vi "Test DB_CONNECTOR API.vi"() -> ()   [LabVIEW 2014]
doc: "DB_CONNECTOR API Tester.\n\n____\nHAMPEL SOFTWARE ENGINEERING v2.4.4 (2020-05-26 17:37)"
uses:
  Query Poly-VIs/Query - String - 2D.vi
  DB_CONNECTOR.lvlib
panel:
  out "DB-Type":string
  in  "Get DB-Type":bool
  in  "btn_Fast_Query":bool caption="btn_Query"
  out "Query Time (ms)":u32
  out "Field Names":string[](array[string])
  in  "Config Section":string
  out "Meta Data":variant
  in  "btn_Commit_Transaction":bool caption="btn_Query"
  in  "btn_Start_Transaction":bool caption="btn_Query"
  out "Return Data":string[][](array[string])
  in  "btn_Query":bool
  in  "SQL Query":string
  in  "Run as Singleton?":bool
  in  "Show Block Diagram":bool
  in  "Refresh Modules":bool
  out "Active Modules":string[](array[string])
  in  "Stop Module":bool
  in  "Select Module":i32(ring)=-1 caption="Select Module\nTo send Request to" items=["All"=-1]
  in  "Run New Module":bool
  in  "Hide Module Panel":bool
  in  "Show Module Panel":bool
  out "Status":string
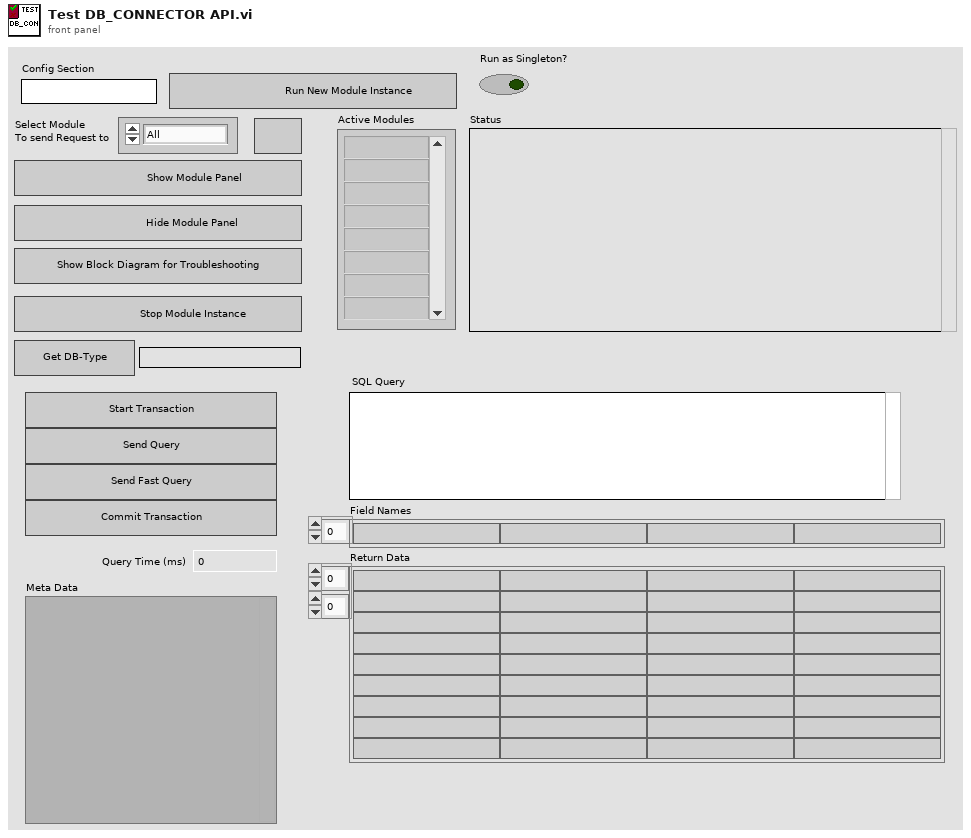
[diagram p1: front panel]
types:
  T1 = typedef "DB_CONNECTOR.lvlib/Broadcast Events--cluster.ctl" = cluster{"Module Did Init":refnum<user-event>, "Status Updated":refnum<user-event>, "Error Reported":refnum<user-event>, "Module Did Stop":refnum<user-event>, "Update Module Execution Status":refnum<user-event>, "Fast Query Reply":refnum<user-event>}
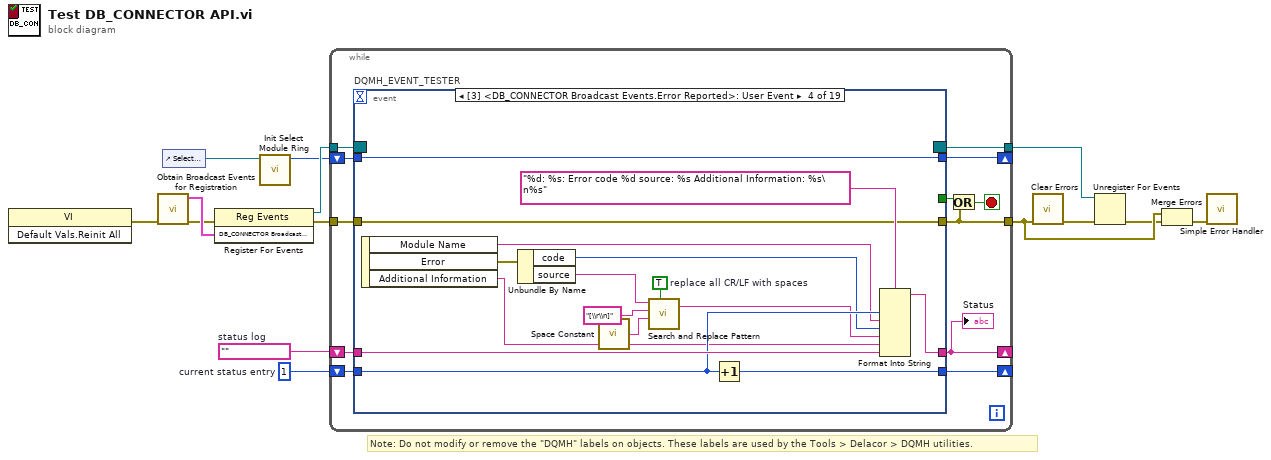
[diagram p0: block diagram]
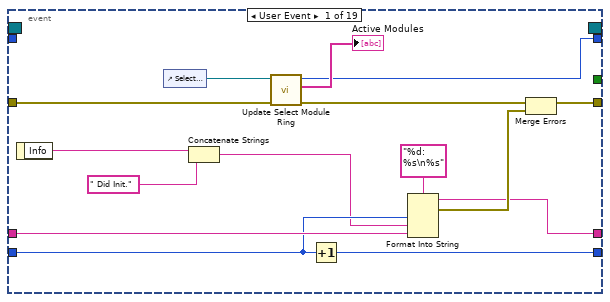
[diagram p2: hidden frame]
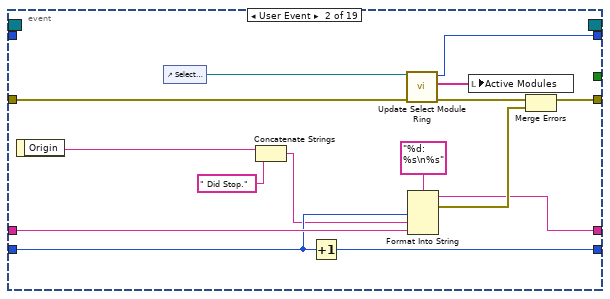
[diagram p3: hidden frame]
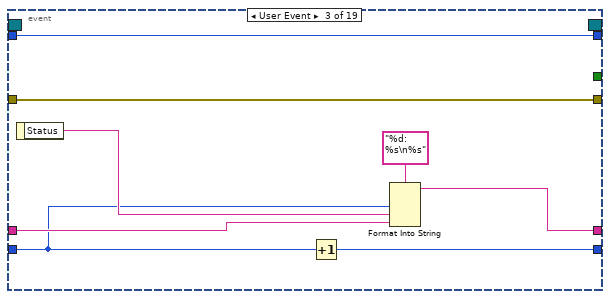
[diagram p4: hidden frame]
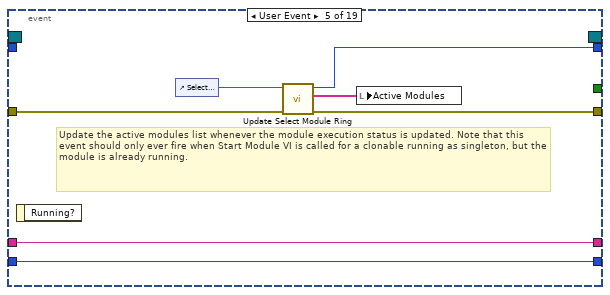
[diagram p5: hidden frame]
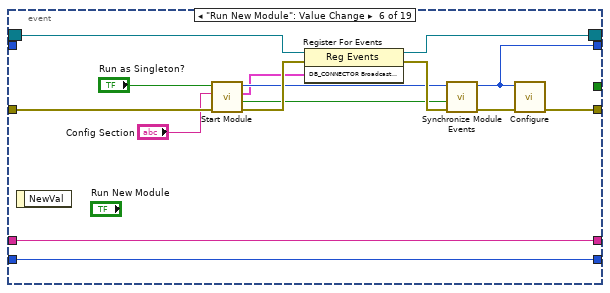
[diagram p6: hidden frame]
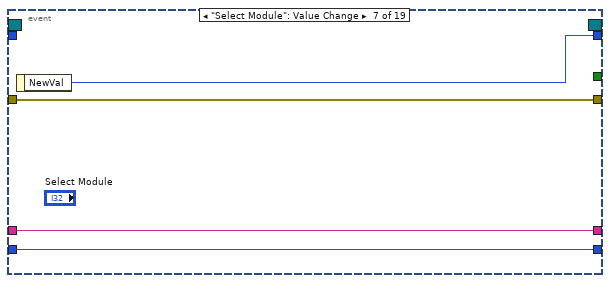
[diagram p7: hidden frame]
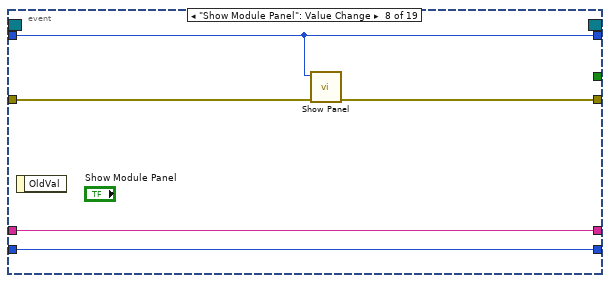
[diagram p8: hidden frame]
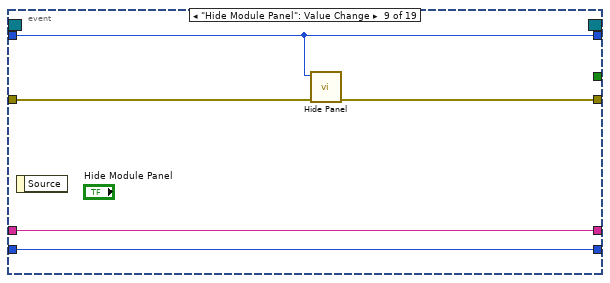
[diagram p9: hidden frame]
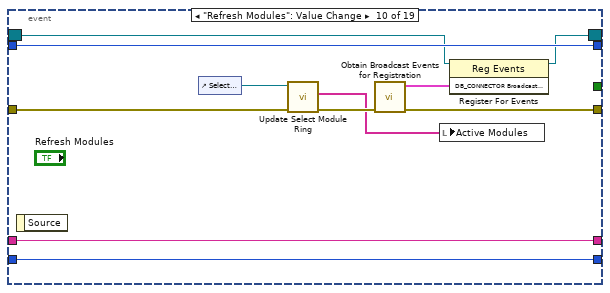
[diagram p10: hidden frame]
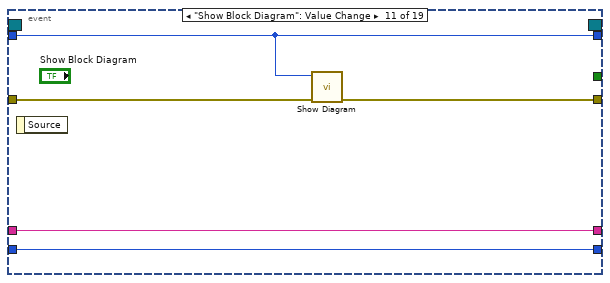
[diagram p11: hidden frame]
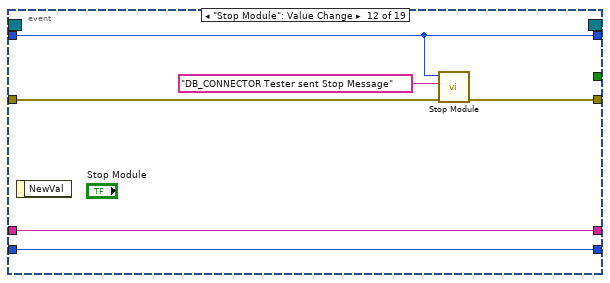
[diagram p12: hidden frame]
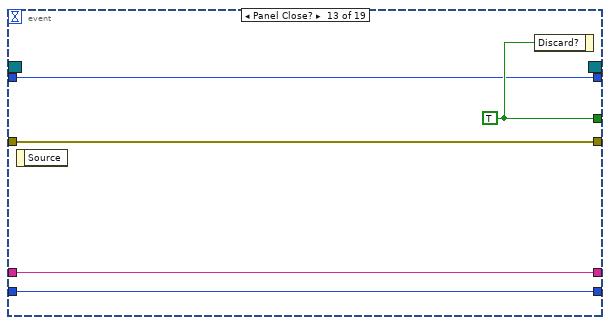
[diagram p13: hidden frame]
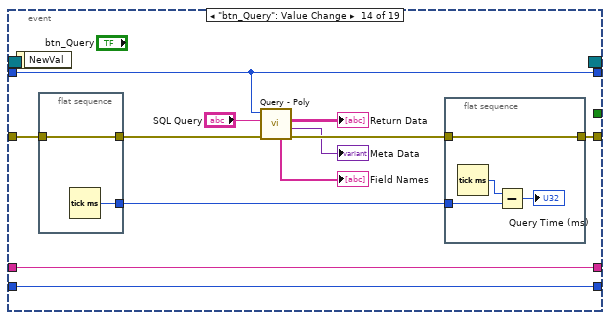
[diagram p14: hidden frame]
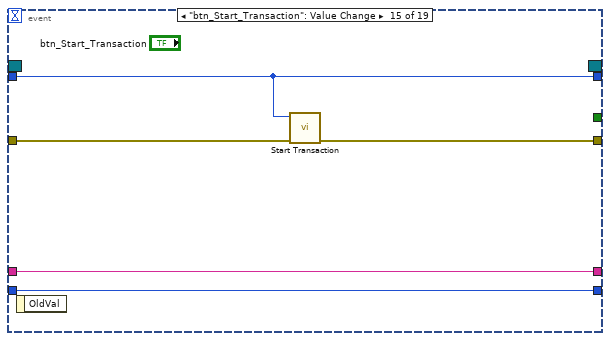
[diagram p15: hidden frame]
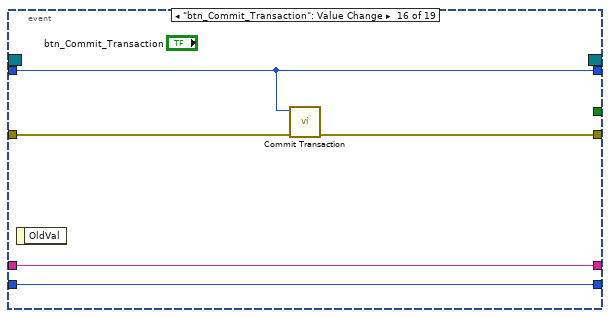
[diagram p16: hidden frame]
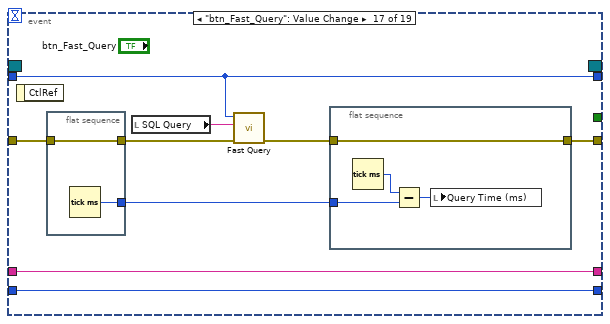
[diagram p17: hidden frame]
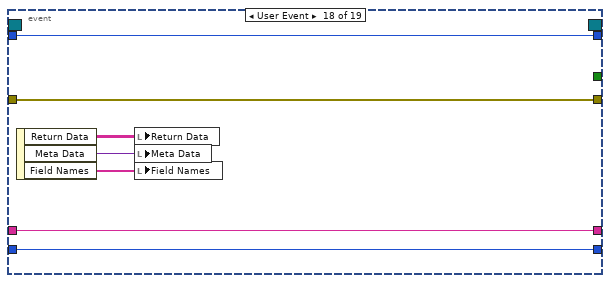
[diagram p18: hidden frame]
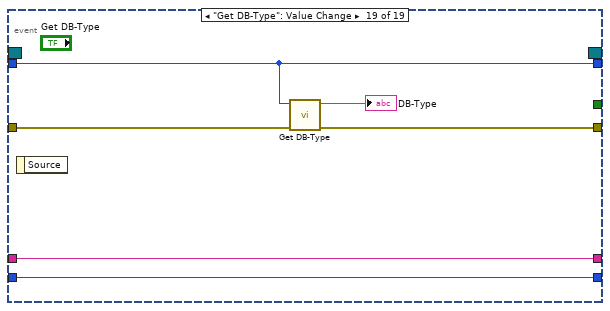
[diagram p19: hidden frame]
diagram:
  w11 = 1  # current status entry
  w12 = ""  # status log
  # "Note: Do not modify or remove the \"DQMH\" labels on objects. These labels are used by the Tools > Delacor > DQMH utilities."
  n1 = invoke class="VI" method="Default Vals.Reinit All"() -> (error out=w3:errorcluster)  [unwired: 3 in, 2 out]
  n2 = call "Obtain Broadcast Events for Registration.vi"("error in (no error)"=w3) -> ("error out"=w2:errorcluster, "DB_CONNECTOR Broadcast Events"=w8:T1)  [unwired: 9 in]
  n3 = control-ref of="Select Module"() -> (w9:refnum<vi>)
  n4 = register-events(error in=w2, w8) -> (reference out=w14:refnum<event-registration>, error out=w7:errorcluster)  [unwired: 1 in]
  n5 = call "Init Select Module Ring.vi"("Select Module Ring Ref"=w9) -> ("Value for All Modules"=w10:i32)  [unwired: 8 in, 2 out]
  n6 = while {
    tunnel: w14 -> [w26]
    tunnel: [w15] -> w4
    tunnel: w7 -> [w24]
    shift-right: [w20] -> _
    shift-left: w12 -> [w22]
    shift-right: [w21] -> _
    shift-left: w11 -> [w23]
    shift-right: [w17] -> _
    shift-left: w10 -> [w18]
    tunnel: [w16] -> w6
    stop <- w19 stop-if-true
    n7 = event "DQMH_EVENT_TESTER" shown="[3] <DB_CONNECTOR Broadcast Events.Error Reported>: User Event" {
      selector: w26 -> [_ _ _ _ _ w97 _ _ _ w122 _ _ _ _ _ _ _ _ _]
      dyn-events: [_ _ _ _ _ w96 _ _ _ w121 _ _ _ _ _ _ _ _ _] -> w16
      timeout: _ -> [_ _ _ _ _ _ _ _ _ _ _ _ _ _ _ _ _ _ _]
      tunnel: [_ _ _ _ _ _ _ _ _ _ _ _ w143 _ _ _ _ _ _] -> w25
      tunnel: [w30 w48 w64 w70 w83 w90 w106 w110 w115 w118 w129 w134 w142 w145 w163 w168 w173 w193 w196] -> w15
      tunnel: w24 -> [w32 w50 w64 w70 w84 w98 w106 w111 w116 w123 w132 w135 w142 w147 w166 w171 w176 w193 w199]
      tunnel: w23 -> [w38 w53 w57 w76 w86 w99 w104 w108 w113 w126 w130 w137 w140 w153 w164 w169 w179 w191 w197]
      tunnel: w22 -> [w39 w54 w60 w78 w87 w100 w105 w109 w114 w127 w131 w138 w141 w154 w165 w170 w180 w192 w198]
      tunnel: [w36 w51 w61 w73 w87 w100 w105 w109 w114 w127 w131 w138 w141 w154 w165 w170 w180 w192 w198] -> w20
      tunnel: [w37 w52 w63 w79 w86 w99 w104 w108 w113 w126 w130 w137 w140 w153 w164 w169 w179 w191 w197] -> w21
      tunnel: w18 -> [_ _ w58 w80 _ _ _ w107 w112 w125 w128 w136 w139 w152 w162 w167 w178 w190 w195]
      tunnel: [w27 w45 w58 w80 w82 w89 w103 w107 w112 w125 w128 w136 w139 w152 w162 w167 w178 w190 w195] -> w17
      event User Event {
        n8 = event-data() -> ("Info"=w35:string)  [unwired: 1 in]
        n9 = control-ref of="Select Module"() -> (w29:refnum<vi>)
        n10 = Concatenate Strings(w35, " Did Init.") -> (w34:string)
        n11 = call "Update Select Module Ring.vi"("error in (no error)"=w32, "Select Module Ring Ref"=w29) -> ("error out"=w31:errorcluster, "Active Modules (Array)"=→"Active Modules":string[], "New Module Ring Value"=w27:i32)  [unwired: 7 in]
        n12 = Increment(x=w38) -> (x+1=w37:i32)
        n13 = Format Into String(format string="%d: %s\n%s", w38, w34, w39) -> (resulting string=w36:string, error out=w41:errorcluster)  [unwired: 2 in]
        n14 = Merge Errors(w31, w41) -> (w30:errorcluster)
      }
      event User Event {
        n15 = event-data() -> ("Origin"=w43:string)  [unwired: 1 in]
        n16 = control-ref of="Select Module"() -> (w47:refnum<vi>)
        n17 = Concatenate Strings(w43, " Did Stop.") -> (w42:string)
        n18 = Increment(x=w53) -> (x+1=w52:i32)
        n19 = call "Update Select Module Ring.vi"("error in (no error)"=w50, "Select Module Ring Ref"=w47) -> ("error out"=w49:errorcluster, "Active Modules (Array)"=w46:string[], "New Module Ring Value"=w45:i32)  [unwired: 7 in]
        n20 = Format Into String(format string="%d: %s\n%s", w53, w42, w54) -> (resulting string=w51:string, error out=w56:errorcluster)  [unwired: 2 in]
        n21 = local write "Active Modules"(w46) -> ()
        n22 = Merge Errors(w49, w56) -> (w48:errorcluster)
      }
      event User Event {
        n23 = event-data() -> ("Status"=w59:string)  [unwired: 1 in]
        n24 = Increment(x=w57) -> (x+1=w63:i32)
        n25 = Format Into String(format string="%d: %s\n%s", w57, w59, w60) -> (resulting string=w61:string)  [unwired: 2 in, 1 out]
      }
      event User Event {
        w74 = TRUE  # replace all CR/LF with spaces
        n26 = event-data() -> ("Module Name"=w68:string, "Error"=w67:errorcluster, "Additional Information"=w65:string)  [unwired: 1 in]
        n27 = Unbundle By Name(w67) -> ("code"=w69:i32, "source"=w71:string)
        n28 = call <vilib>:"Space Constant.vi"() -> ("String"=w75:string)
        n29 = call <vilib>:"Search and Replace Pattern.vi"("string"=w71, "regular expression (\"\")"="[\\r\\n]" ("regular expression (\"\")"), "replace string (\"\")"=w75, "replace all? (F)"=w74) -> ("result string"=w72:string)  [unwired: 1 in, 1 out]
        n30 = Increment(x=w76) -> (x+1=w79:i32)
        n31 = Format Into String(format string="%d: %s: Error code %d source: %s Additional Information: %s\n%s", w76, w68, w69, w72, w65, w78) -> (resulting string=w73:string)  [unwired: 2 in, 1 out]
      }
      event User Event {
        # "Update the active modules list whenever the module execution status is updated. Note that this event should only ever fire when Start Module VI is called for a clonable running as singleton, but the module is already running."
        n32 = event-data() -> ()  [unwired: 1 in, 1 out]
        n33 = control-ref of="Select Module"() -> (w85:refnum<vi>)
        n34 = call "Update Select Module Ring.vi"("error in (no error)"=w84, "Select Module Ring Ref"=w85) -> ("error out"=w83:errorcluster, "Active Modules (Array)"=w81:string[], "New Module Ring Value"=w82:i32)  [unwired: 7 in]
        n35 = local write "Active Modules"(w81) -> ()
      }
      event "Run New Module": Value Change {
        n36 = event-data() -> ()  [unwired: 1 in, 1 out]
        n37 = call "Start Module.vi"("error in (no error)"=w98, "Config Section"="Config Section", "Run as Singleton? (F)"="Run as Singleton?") -> ("error out"=w101:errorcluster, "Wait for Event Sync?"=w94:bool, "DB_CONNECTOR Broadcast Events"=w93:T1, "Module ID"=w95:i32)  [unwired: 5 in]
        n38 = register-events(reference=w97, error in=w101, w93) -> (reference out=w96:refnum<event-registration>, error out=w102:errorcluster)
        n39 = call "Synchronize Module Events.vi"("error in (no error)"=w102, "Wait for Event Sync?"=w94, "Module ID"=w95) -> ("error out"=w91:errorcluster, "Module ID (dup)"=w89:i32)  [unwired: 7 in]
        n40 = call "Configure.vi"("error in (no error)"=w91, "Module ID"=w89) -> ("error out"=w90:errorcluster)  [unwired: 8 in, 1 out]
      }
      event "Select Module": Value Change {
        n41 = event-data() -> ("NewVal"=w103:i32)  [unwired: 1 in]
      }
      event "Show Module Panel": Value Change {
        n42 = event-data() -> ()  [unwired: 1 in, 1 out]
        n43 = call "Show Panel.vi"("error in (no error)"=w111, "Module ID"=w107) -> ("error out"=w110:errorcluster)  [unwired: 9 in]
      }
      event "Hide Module Panel": Value Change {
        n44 = event-data() -> ()  [unwired: 1 in, 1 out]
        n45 = call "Hide Panel.vi"("error in (no error)"=w116, "Module ID"=w112) -> ("error out"=w115:errorcluster)  [unwired: 9 in]
      }
      event "Refresh Modules": Value Change {
        n46 = event-data() -> ()  [unwired: 1 in, 1 out]
        n47 = control-ref of="Select Module"() -> (w124:refnum<vi>)
        n48 = call "Update Select Module Ring.vi"("error in (no error)"=w123, "Select Module Ring Ref"=w124) -> ("error out"=w119:errorcluster, "Active Modules (Array)"=w117:string[])  [unwired: 7 in, 1 out]
        n49 = call "Obtain Broadcast Events for Registration.vi"("error in (no error)"=w119) -> ("error out"=w118:errorcluster, "DB_CONNECTOR Broadcast Events"=w120:T1)  [unwired: 9 in]
        n50 = local write "Active Modules"(w117) -> ()
        n51 = register-events(reference=w122, w120) -> (reference out=w121:refnum<event-registration>)  [unwired: 1 in, 1 out]
      }
      event "Show Block Diagram": Value Change {
        n52 = event-data() -> ()  [unwired: 1 in, 1 out]
        n53 = call "Show Diagram.vi"("error in (no error)"=w132, "Module ID"=w128) -> ("error out"=w129:errorcluster)  [unwired: 9 in]
      }
      event "Stop Module": Value Change {
        n54 = event-data() -> ()  [unwired: 1 in, 1 out]
        n55 = call "Stop Module.vi"("error in (no error)"=w135, "Origin"="DB_CONNECTOR Tester sent Stop Message", "Module ID"=w136) -> ("error out"=w134:errorcluster)  [unwired: 8 in]
      }
      event Panel Close? {
        w143 = TRUE ("Discard?")
        n56 = event-data() -> ()  [unwired: 1 in, 1 out]
        n57 = event-data("Discard?"=w143) -> ()  [unwired: 1 in, 1 out]
      }
      event "btn_Query": Value Change {
        n58 = event-data() -> ()  [unwired: 1 in, 1 out]
        n59 = flat-sequence {
          tunnel: w147 -> [w161]
          tunnel: [w161] -> w146
          tunnel: [w160] -> w144
          frame #0 {
            n60 = Tick Count (ms)() -> (millisecond timer value=w160:u32)
          }
        }
        n61 = call-poly "Query - Poly.vi"("error in"=w146, "Query"="SQL Query", "Module ID"=w152) -> ("error out"=w155:errorcluster, "Meta Data"=→"Meta Data":variant, "Return Data"=→"Return Data":string[][], "Field Names"=→"Field Names":string[])  [unwired: 5 in]
        n62 = flat-sequence {
          tunnel: w155 -> [w159]
          tunnel: [w159] -> w145
          tunnel: w144 -> [w157]
          frame #0 {
            n63 = Tick Count (ms)() -> (millisecond timer value=w158:u32)
            n64 = Subtract(x=w158, y=w157) -> (x-y=→"Query Time (ms)":u32)
          }
        }
      }
      event "btn_Start_Transaction": Value Change {
        n65 = event-data() -> ()  [unwired: 1 in, 1 out]
        n66 = call "Start Transaction.vi"("error in (no error)"=w166, "Module ID"=w162) -> ("error out"=w163:errorcluster)  [unwired: 9 in]
      }
      event "btn_Commit_Transaction": Value Change {
        n67 = event-data() -> ()  [unwired: 1 in, 1 out]
        n68 = call "Commit Transaction.vi"("error in (no error)"=w171, "Module ID"=w167) -> ("error out"=w168:errorcluster)  [unwired: 7 in, 2 out]
      }
      event "btn_Fast_Query": Value Change {
        n69 = event-data() -> ()  [unwired: 1 in, 1 out]
        n70 = flat-sequence {
          tunnel: w176 -> [w186]
          tunnel: [w186] -> w175
          tunnel: [w185] -> w172
          frame #0 {
            n71 = Tick Count (ms)() -> (millisecond timer value=w185:u32)
          }
        }
        n72 = local read "SQL Query"() -> (w177:string)
        n73 = call "Fast Query.vi"("error in (no error)"=w175, "Query"=w177, "Module ID"=w178) -> ("error out"=w174:errorcluster)  [unwired: 8 in]
        n74 = flat-sequence {
          tunnel: w174 -> [w184]
          tunnel: [w184] -> w173
          tunnel: w172 -> [w182]
          frame #0 {
            n75 = Tick Count (ms)() -> (millisecond timer value=w183:u32)
            n76 = Subtract(x=w183, y=w182) -> (x-y=w181:u32)
            n77 = local write "Query Time (ms)"(w181) -> ()
          }
        }
      }
      event User Event {
        n78 = event-data() -> ("Return Data"=w189:string[][], "Meta Data"=w188:variant, "Field Names"=w187:string[])  [unwired: 1 in]
        n79 = local write "Return Data"(w189) -> ()
        n80 = local write "Meta Data"(w188) -> ()
        n81 = local write "Field Names"(w187) -> ()
      }
      event "Get DB-Type": Value Change {
        n82 = event-data() -> ()  [unwired: 1 in, 1 out]
        n83 = call "Get DB-Type.vi"("error in (no error)"=w199, "Module ID"=w195) -> ("error out"=w196:errorcluster, "DB-Type"=→"DB-Type":string)  [unwired: 8 in]
      }
    }
    "Status" <- w20
    n84 = Or(x=w25, y=w15) -> (x .or. y?=w19:bool)
  }
  n85 = call <vilib>:"Clear Errors.vi"("error in (no error)"=w4) -> ("error out"=w13:errorcluster)  [unwired: 5 in, 1 out]
  n86 = Unregister For Events(event registration refnum=w6, error in=w13) -> (error out=w1:errorcluster)
  n87 = Merge Errors(w4, w1) -> (w5:errorcluster)
  n88 = call <vilib>:"Simple Error Handler.vi"("error in (no error)"=w5) -> ()  [unwired: 4 in, 5 out]
